vi "XIPIN_AXI4-Stream_Interconnect_RTL_1_1.vi"   [LabVIEW 2017]
doc: "The AXI4-Stream Interconnect IP provides the infrastructure to connect multiple AXI4-Stream masters and slaves. The configurable interconnect features a 16x16 switch, data FIFOs, register slices, data width converters and clock rate converters.\n------------------------------------\n<b>Need License</b> : No\n<b>Interface</b> : AXI4-Stream"
uses:
  <vilib>/rvi/XilinxIP/XIPIN_XNode/niFpgaXIPIN.xnode
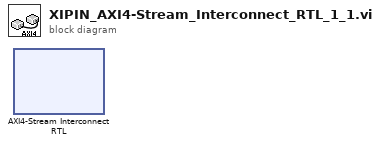
[diagram p0: block diagram]
diagram:
  n1 = xnode ("AXI4-Stream Interconnect RTL")() -> ()
